vi "Dew_point_measurement_(DMT143)_v1.vi"() -> ()   [LabVIEW 2018]
uses:
  <vilib>/Instr/_visa.llb/VISA Configure Serial Port (Instr).vi
panel:
  in  "Clear Graphs":bool
  out "read buffer":string
  in  "Grid on/off":enum32{"Radio Selection 1", "Radio Selection 2"}(radio)=enum."Radio Selection 2"
  in  "Save":bool
  in  "File name":string="Name"
  in  "Delay [ms]":u32=1000
  out "RH":cluster{dbl, "H":dbl}[](graph)
  out "RH":dbl format="%#_4g"
  out "H2O[ppm]":cluster{dbl, dbl}[](graph)
  out "Dew-Point['C]":cluster{dbl, dbl}[](graph)
  in  "stop":bool
  out "H2O[ppm]":string
  out "Tdfatm['C]":string
  out "Tdf['C]":string
  in  "COM port":refnum<visa-resource-name>="COM9"
  # "%"
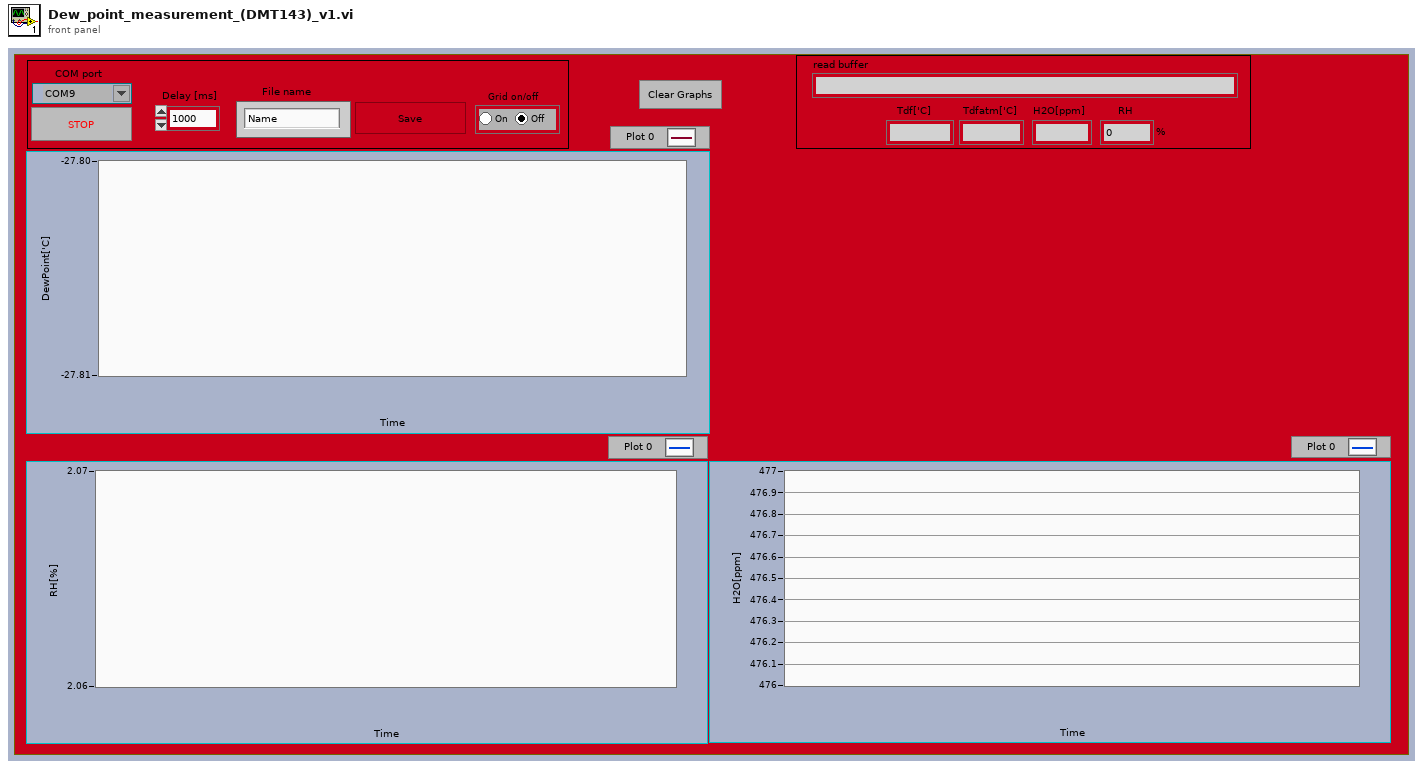
[diagram p1: front panel]
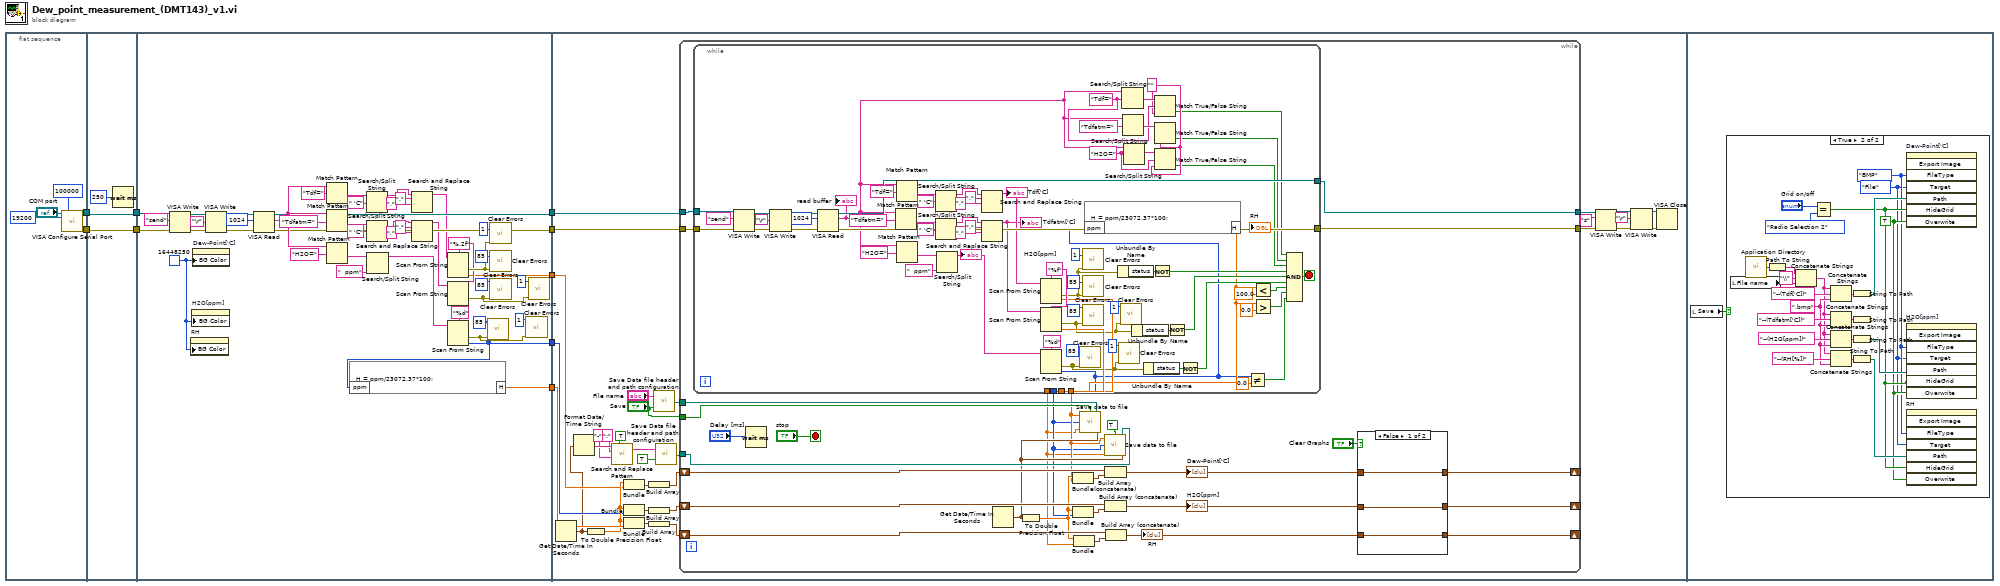
[diagram p0: block diagram]
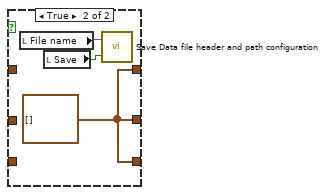
[diagram p2: hidden frame]
diagram:
  n1 = flat-sequence {
    tunnel: [w12] -> w9
    tunnel: [w11] -> w8
    tunnel: [w15] -> w5
    tunnel: [w16] -> w7
    tunnel: w9 -> [w15]
    tunnel: w8 -> [w16]
    tunnel: w7 -> [w32]
    tunnel: [w30] -> w6
    tunnel: w5 -> [w33]
    tunnel: [w31] -> w4
    tunnel: [w28] -> w3
    tunnel: [w26] -> w2
    tunnel: [w27] -> w1
    tunnel: w6 -> [w84]
    tunnel: w4 -> [w85]
    tunnel: w3 -> [w77]
    tunnel: w2 -> [w76]
    tunnel: w1 -> [w81]
    frame #0 {
      n2 = call-poly "VISA Configure Serial Port"("VISA resource name"="COM port", "timeout (10sec)"=u32 100000, "baud rate (9600)"=u32 19200) -> ("VISA resource name out"=w12:refnum<visa-resource-name>, "error out"=w11:errorcluster)  [unwired: 11 in]
    }
    frame #1 {
      n3 = Wait (ms)(milliseconds to wait=u32 250) -> ()  [unwired: 1 out]
    }
    frame #2 {
      w29 = u32 16448250
      w52 = "%.2f" ("format string")
      n4 = VISA Write(VISA resource name=w33, write buffer="send", error in (no error)=w32) -> (VISA resource name out=w41:refnum<visa-resource-name>, error out=w40:errorcluster)  [unwired: 1 out]
      n5 = property on="RH" class="XYGraph (strict)"("BG Color"=w29) -> ()  [unwired: 2 in, 2 out]
      n6 = property on="H2O[ppm]" class="XYGraph (strict)"("BG Color"=w29) -> ()  [unwired: 2 in, 2 out]
      n7 = property on="Dew-Point['C]" class="XYGraph (strict)"("BG Color"=w29) -> ()  [unwired: 2 in, 2 out]
      n8 = VISA Write(VISA resource name=w41, write buffer="\r", error in (no error)=w40) -> (VISA resource name out=w39:refnum<visa-resource-name>, error out=w38:errorcluster)  [unwired: 1 out]
      n9 = VISA Read(VISA resource name=w39, byte count=u32 1024, error in (no error)=w38) -> (VISA resource name out=w31:refnum<visa-resource-name>, read buffer=w34:string, error out=w30:errorcluster)  [unwired: 1 out]
      n10 = Match Pattern(string=w34, regular expression="Tdfatm=" ("search string/char (-)")) -> (after substring=w35:string)  [unwired: 1 in, 3 out]
      n11 = Match Pattern(string=w34, regular expression="Tdf=" ("search string/char (-)")) -> (after substring=w37:string)  [unwired: 1 in, 3 out]
      n12 = Match Pattern(string=w34, regular expression="H2O=" ("search string/char (-)")) -> (after substring=w36:string)  [unwired: 1 in, 3 out]
      n13 = Search/Split String(string=w37, search string/char (-)=" 'C") -> (substring before match=w23:string)  [unwired: 1 in, 2 out]
      n14 = Search/Split String(string=w35, search string/char (-)=" 'C") -> (substring before match=w19:string)  [unwired: 1 in, 2 out]
      n15 = Search/Split String(string=w36, search string/char (-)="  ppm") -> (substring before match=w51:string)  [unwired: 1 in, 2 out]
      n16 = Search and Replace String(input string=w23, search string=".", replace string="," ("search string")) -> (result string=w22:string)  [unwired: 5 in, 3 out]
      n17 = Search and Replace String(input string=w19, search string=".", replace string="," ("search string")) -> (result string=w18:string)  [unwired: 5 in, 3 out]
      n18 = Scan From String(format string=w52, input string=w22) -> (error out=w58:errorcluster, output 1=w28:dbl)  [unwired: 3 in, 2 out]
      n19 = Scan From String(format string=w52, input string=w18) -> (error out=w60:errorcluster)  [unwired: 4 in, 2 out]
      n20 = Scan From String(format string="%d", input string=w51) -> (error out=w62:errorcluster, output 1=w26:i32)  [unwired: 3 in, 2 out]
      n21 = formula code="H = ppm/23072.37*100;"("ppm"=w26) -> ("H"=w27:dbl)
      n22 = call <vilib>:"Clear Errors.vi"("error in (no error)"=w62, "specific error code to clear (0: all)"=85) -> ()  [unwired: 4 in, 2 out]
      n23 = call <vilib>:"Clear Errors.vi"("error in (no error)"=w58, "specific error code to clear (0: all)"=1) -> ()  [unwired: 4 in, 2 out]
      n24 = call <vilib>:"Clear Errors.vi"("error in (no error)"=w58, "specific error code to clear (0: all)"=85) -> ()  [unwired: 4 in, 2 out]
      n25 = call <vilib>:"Clear Errors.vi"("error in (no error)"=w60, "specific error code to clear (0: all)"=85) -> ()  [unwired: 4 in, 2 out]
      n26 = call <vilib>:"Clear Errors.vi"("error in (no error)"=w62, "specific error code to clear (0: all)"=1) -> ()  [unwired: 4 in, 2 out]
      n27 = call <vilib>:"Clear Errors.vi"("error in (no error)"=w60, "specific error code to clear (0: all)"=1) -> ()  [unwired: 4 in, 2 out]
    }
    frame #3 {
      n28 = Get Date/Time In Seconds() -> (seconds since 1Jan1904=w69:timestamp)
      n29 = Format Date/Time String(seconds (now)=w69) -> (date/time string=w73:string)  [unwired: 2 in]
      n30 = To Double Precision Float(number=w69) -> (double precision float=w79:dbl)
      n31 = call <vilib>:"Search and Replace Pattern.vi"("string"=w73, "regular expression (\"\")"=":" ("regular expression (\"\")"), "replace string (\"\")"="-" ("replace string (\"\")"), "replace all? (F)"=TRUE) -> ("result string"=w64:string)  [unwired: 1 in, 1 out]
      n32 = Bundle(w79, w77) -> (w80:cluster{dbl, dbl})  [unwired: 1 in]
      n33 = Bundle(w79, w76) -> (w75:cluster{dbl, i32})  [unwired: 1 in]
      n34 = Bundle(w79, "H"=w81) -> (w82:cluster{dbl, "H":dbl})  [unwired: 1 in]
      n35 = Build Array(w80) -> (w78:cluster{dbl, dbl}[])
      n36 = Build Array(w75) -> (w74:cluster{dbl, i32}[])
      n37 = Build Array(w82) -> (w83:cluster{dbl, "H":dbl}[])
      n38 = call "Save Data file header and path configuration.vi"("Save"="Save", "File name"="File name") -> ("Output Path"=w66:path)
      n39 = call "Save Data file header and path configuration.vi"("Save"=TRUE, "File name"=w64) -> ("Output Path"=w63:path)
      n40 = while {
        tunnel: w85 -> [w111]
        tunnel: w84 -> [w110]
        shift-right: [w107] -> _
        shift-left: w78 -> [w120]
        shift-right: [w105] -> _
        shift-left: w74 -> [w118]
        tunnel: [w109] -> w93
        tunnel: [w116] -> w92
        shift-right: [w103] -> _
        shift-left: w83 -> [w114]
        tunnel: w66 -> [w99]
        tunnel: "Save" -> [w98]
        tunnel: w63 -> [w100]
        stop <- "stop" stop-if-true
        n41 = while {
          tunnel: [w166] -> _
          tunnel: [w136] -> w95
          tunnel: [w141] -> w94
          tunnel: w111 -> [w179]
          tunnel: [w168] -> w109
          tunnel: w110 -> [w178]
          tunnel: [w167] -> w116
          tunnel: [w165] -> w96
          stop <- w155 stop-if-true
          w151 = "Tdf=" ("true string")
          w150 = "" ("false string")
          w149 = "H2O=" ("true string")
          w148 = "Tdfatm=" ("true string")
          w176 = "%f" ("format string")
          n42 = VISA Write(VISA resource name=w179, write buffer="send", error in (no error)=w178) -> (VISA resource name out=w189:refnum<visa-resource-name>, error out=w190:errorcluster)  [unwired: 1 out]
          n43 = VISA Write(VISA resource name=w189, write buffer="\r", error in (no error)=w190) -> (VISA resource name out=w191:refnum<visa-resource-name>, error out=w192:errorcluster)  [unwired: 1 out]
          n44 = VISA Read(VISA resource name=w191, byte count=u32 1024, error in (no error)=w192) -> (VISA resource name out=w168:refnum<visa-resource-name>, read buffer=w147:string, error out=w167:errorcluster)  [unwired: 1 out]
          "read buffer" <- w147
          n45 = Match Pattern(string=w147, regular expression="Tdfatm=" ("search string/char (-)")) -> (after substring=w195:string)  [unwired: 1 in, 3 out]
          n46 = Match Pattern(string=w147, regular expression="Tdf=" ("search string/char (-)")) -> (after substring=w193:string)  [unwired: 1 in, 3 out]
          n47 = Match Pattern(string=w147, regular expression="H2O=" ("search string/char (-)")) -> (after substring=w194:string)  [unwired: 1 in, 3 out]
          n48 = Search/Split String(string=w193, search string/char (-)=" 'C") -> (substring before match=w131:string)  [unwired: 1 in, 2 out]
          n49 = Search/Split String(string=w195, search string/char (-)=" 'C") -> (substring before match=w129:string)  [unwired: 1 in, 2 out]
          n50 = Search/Split String(string=w194, search string/char (-)="  ppm") -> (substring before match=w177:string)  [unwired: 1 in, 2 out]
          "H2O[ppm]" <- w177
          n51 = Search and Replace String(input string=w131, search string=".", replace string="," ("search string")) -> (result string=w130:string)  [unwired: 5 in, 3 out]
          "Tdf['C]" <- w130
          n52 = Search and Replace String(input string=w129, search string=".", replace string="," ("search string")) -> (result string=w128:string)  [unwired: 5 in, 3 out]
          "Tdfatm['C]" <- w128
          n53 = Scan From String(format string=w176, input string=w130) -> (error out=w164:errorcluster, output 1=w165:dbl)  [unwired: 3 in, 2 out]
          n54 = Scan From String(format string=w176, input string=w128) -> (error out=w163:errorcluster, output 1=w166:dbl)  [unwired: 3 in, 2 out]
          n55 = Scan From String(format string="%d", input string=w177) -> (error out=w162:errorcluster, output 1=w136:i32)  [unwired: 3 in, 2 out]
          n56 = call <vilib>:"Clear Errors.vi"("error in (no error)"=w162, "specific error code to clear (0: all)"=85) -> ()  [unwired: 4 in, 2 out]
          n57 = call <vilib>:"Clear Errors.vi"("error in (no error)"=w164, "specific error code to clear (0: all)"=1) -> ()  [unwired: 4 in, 2 out]
          n58 = call <vilib>:"Clear Errors.vi"("error in (no error)"=w164, "specific error code to clear (0: all)"=85) -> ()  [unwired: 4 in, 2 out]
          n59 = call <vilib>:"Clear Errors.vi"("error in (no error)"=w163, "specific error code to clear (0: all)"=85) -> ()  [unwired: 4 in, 2 out]
          n60 = formula code="H = ppm/23072.37*100;"("ppm"=w136) -> ("H"=w141:dbl)
          "RH" <- w141
          n61 = Unbundle By Name(w164) -> ("status"=w161:bool)
          n62 = call <vilib>:"Clear Errors.vi"("error in (no error)"=w162, "specific error code to clear (0: all)"=1) -> ()  [unwired: 4 in, 2 out]
          n63 = call <vilib>:"Clear Errors.vi"("error in (no error)"=w163, "specific error code to clear (0: all)"=1) -> ()  [unwired: 4 in, 2 out]
          n64 = Search/Split String(string=w147, search string/char (-)=w151) -> (match + rest of string=w152:string)  [unwired: 1 in, 2 out]
          n65 = Search/Split String(string=w147, search string/char (-)=w148) -> (match + rest of string=w154:string)  [unwired: 1 in, 2 out]
          n66 = Search/Split String(string=w147, search string/char (-)=w149) -> (match + rest of string=w153:string)  [unwired: 1 in, 2 out]
          n67 = Unbundle By Name(w163) -> ("status"=w160:bool)
          n68 = Unbundle By Name(w162) -> ("status"=w159:bool)
          n69 = Not(x=w161) -> (.not. x?=w158:bool)
          n70 = Match True/False String(2:w150, 3:w151, 4:w152) -> (0:w144:bool)  [unwired: 1 out]
          n71 = Match True/False String(2:w150, 3:w148, 4:w154) -> (0:w145:bool)  [unwired: 1 out]
          n72 = Match True/False String(2:w150, 3:w149, 4:w153) -> (0:w146:bool)  [unwired: 1 out]
          n73 = Not(x=w160) -> (.not. x?=w157:bool)
          n74 = Not(x=w159) -> (.not. x?=w156:bool)
          n75 = Not Equal?(x=w136, y=0.0) -> (x != y?=w137:bool)
          n76 = Less?(x=w141, y=100.0) -> (x < y?=w140:bool)
          n77 = Greater?(x=w141, y=0.0) -> (0:w139:bool)
          n78 = Compound Arithmetic op=AND(w144, w145, w146, w158, w157, w156, w140, w139, w137) -> (w155:bool)
        }
        n79 = Wait (ms)(milliseconds to wait="Delay [ms]") -> ()  [unwired: 1 out]
        n80 = Get Date/Time In Seconds() -> (seconds since 1Jan1904=w97:timestamp)
        n81 = To Double Precision Float(number=w97) -> (double precision float=w113:dbl)
        n82 = Bundle(w113, w96) -> (w119:cluster{dbl, dbl})  [unwired: 1 in]
        n83 = Bundle(w113, w95) -> (w117:cluster{dbl, i32})  [unwired: 1 in]
        n84 = Bundle(w113, "H"=w94) -> (w115:cluster{dbl, "H":dbl})  [unwired: 1 in]
        n85 = call "Save data to file.vi"("current time"=w97, "Save path"=w99, "Save"=w98, "RH"=w94, "H2O[ppm]"=w95, "Tdf['C]"=w96) -> ()
        n86 = call "Save data to file.vi"("current time"=w97, "Save path"=w100, "Save"=TRUE, "RH"=w94, "H2O[ppm]"=w95, "Tdf['C]"=w96) -> ()
        n87 = Build Array (concatenate)(w120, w119) -> (w108:cluster{dbl, dbl}[])
        "Dew-Point['C]" <- w108
        n88 = Build Array (concatenate)(w118, w117) -> (w106:cluster{dbl, dbl}[])
        "H2O[ppm]" <- w106
        n89 = Build Array (concatenate)(w114, w115) -> (w104:cluster{dbl, "H":dbl}[])
        "RH" <- w104
        n90 = case shown="False" "Clear Graphs" {
          tunnel: w108 -> [w124 _]
          tunnel: [w124 w127] -> w107
          tunnel: [w123 w127] -> w105
          tunnel: w106 -> [w123 _]
          tunnel: w104 -> [w122 _]
          tunnel: [w122 w127] -> w103
          frame False {
          }
          frame True {
            w127 = cluster{dbl, dbl}[] []
            n91 = local read "File name"() -> (w126:string)
            n92 = local read "Save"() -> (w125:bool)
            n93 = call "Save Data file header and path configuration.vi"("Save"=w125, "File name"=w126) -> ()  [unwired: 1 out]
          }
        }
      }
      n94 = VISA Write(VISA resource name=w93, write buffer="s", error in (no error)=w92) -> (VISA resource name out=w89:refnum<visa-resource-name>, error out=w88:errorcluster)  [unwired: 1 out]
      n95 = VISA Write(VISA resource name=w89, write buffer="\r", error in (no error)=w88) -> (VISA resource name out=w87:refnum<visa-resource-name>, error out=w86:errorcluster)  [unwired: 1 out]
      n96 = VISA Close(VISA resource name=w87, error in (no error)=w86) -> ()  [unwired: 1 out]
    }
    frame #4 {
      n97 = local read "Save"() -> (w196:bool)
      n98 = case shown="True" w196 {
        frame False {
        }
        frame True {
          w205 = ".bmp" ("string")
          w198 = enum32{"BMP", "EPS", "EMF", "PICT"}."BMP" ("File Type")
          w197 = enum32{"File", "Clipboard"}."File" ("Target")
          w199 = TRUE ("Hide Grid")
          n99 = local read "File name"() -> (w216:string)
          n100 = call <vilib>:"Application Directory.vi"() -> ("Application Directory"=w218:path)
          n101 = Path To String(path=w218) -> (string=w219:string)
          n102 = Concatenate Strings(w219, "\\" ("string"), w216) -> (w204:string)
          n103 = Equal?(x="Grid on/off", y=enum32{"Radio Selection 1", "Radio Selection 2"}."Radio Selection 2") -> (x = y?=w200:bool)
          n104 = Concatenate Strings(w204, "--(Tdf['C])" ("string"), w205) -> (w213:string)
          n105 = Concatenate Strings(w204, "--(Tdfatm['C])" ("string"), w205) -> (w212:string)
          n106 = Concatenate Strings(w204, "--(H2O[ppm])" ("string"), w205) -> (w209:string)
          n107 = Concatenate Strings(w204, "--(RH[%])" ("string"), w205) -> (w206:string)
          n108 = String To Path(string=w213) -> (path=w203:path)
          n109 = String To Path(string=w212) -> ()  [unwired: 1 out]
          n110 = String To Path(string=w209) -> (path=w202:path)
          n111 = String To Path(string=w206) -> (path=w201:path)
          n112 = invoke on="Dew-Point['C]" class="XYGraph (strict)" method="Export Image"("FileType"=w198, "Target"=w197, "Path"=w203, "HideGrid"=w200, "Overwrite"=w199) -> ()  [unwired: 3 in, 8 out]
          n113 = invoke on="H2O[ppm]" class="XYGraph (strict)" method="Export Image"("FileType"=w198, "Target"=w197, "Path"=w202, "HideGrid"=w200, "Overwrite"=w199) -> ()  [unwired: 3 in, 8 out]
          n114 = invoke on="RH" class="XYGraph (strict)" method="Export Image"("FileType"=w198, "Target"=w197, "Path"=w201, "HideGrid"=w200, "Overwrite"=w199) -> ()  [unwired: 3 in, 8 out]
        }
      }
    }
  }
